vi "Rect_to_ROI.vi"(0 "rect":T1, 1 "binning":cluster{"x":u8, "y":u8}={"x"=1, "y"=1}) -> (2 "ROI":T2 {"Contours"."Type" items=["No Selection", "Point", "Line", "Rectangle", "Oval", "Polygon", "Freehand Region", "Annulus", "Unused2", "Unused3", "Broken Line", "Freehand Line", "Rotated Rectangle"]})   [LabVIEW 2010]
uses:
  <userlib>/bias2/subvis/ROI_rect.ctl
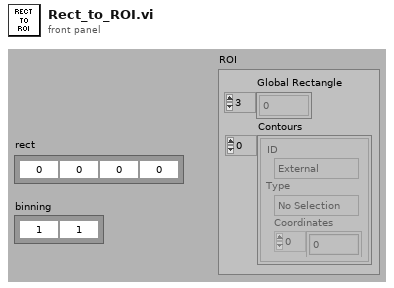
[diagram p1: front panel]
types:
  T1 = typedef "ROI_rect.ctl" = cluster{"left":i32, "top":i32, "right":i32, "bottom":i32}
  T2 = typedef "ROI Descriptor" = cluster{"Global Rectangle":i32[], "Contours":cluster{"ID":enum32{"External", "Internal"}, "Type":u32, "Coordinates":i32[]}[]}
  T3 = cluster{"ID":enum32{"External", "Internal"}, "Type":u32, "rect":i32[]}
  T4 = cluster{"ID":enum32{"External", "Internal"}, "Type":u32, "rect":i32[]}[]
  T5 = cluster{"rect":i32[], cluster{"ID":enum32{"External", "Internal"}, "Type":u32, "rect":i32[]}[]}
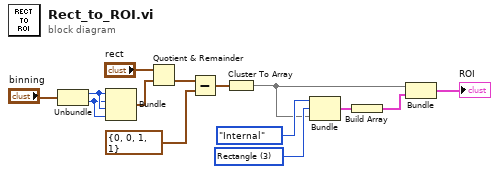
[diagram p0: block diagram]
diagram:
  w13 = u32 3 items=["No Selection", "Point", "Line", "Rectangle", "Oval", "Polygon", "Freehand Region", "Annulus", "Unused2", "Unused3", "Broken Line", "Freehand Line", "Rotated Rectangle"] ("Type")
  n1 = Unbundle("binning") -> ("x"=w8:u8, "y"=w7:u8)
  n2 = Bundle("x"=w8, "y"=w7, "x"=w8, "y"=w7) -> (w5:cluster{"x":u8, "y":u8, "x":u8, "y":u8})  [unwired: 1 in]
  n3 = Quotient & Remainder(x="rect", y=w5) -> (floor(x/y)=w1:T1)  [unwired: 1 out]
  n4 = Subtract(x=w1, y=T1 {"left"=0, "top"=0, "right"=1, "bottom"=1} ("rect 2")) -> (x-y=w3:T1)
  n5 = Cluster To Array(cluster=w3) -> (array=w2:i32[])
  n6 = Bundle("ID"=enum32{"External", "Internal"}."Internal", "Type"=w13, "rect"=w2) -> (w12:T3)  [unwired: 1 in]
  n7 = Build Array(w12) -> (w11:T4)
  n8 = Bundle("rect"=w2, w11) -> (→"ROI":T5)  [unwired: 1 in]
